vi "Тест_буфера_дублирвание_строк.vi"() -> ()   [LabVIEW 2013]
panel:
  out "Исходное сообщение":dbl[](array[numeric])
  in  "Кол-во копий":i32=5
  out "Подготовленный к отправке мажоритарный код":dbl[][](array[numeric])
  out "2-х массив на выходе 3":dbl[][](array[numeric])
  in  "Размер окна":i32=4
  out "Последовательность в массиве":dbl[](array[numeric])
  in  "Кол-во элементов":i32=16
  out "Array":dbl[][](array[numeric])
  in  "Размер окна буффера":i32
  out "Количество бит":i32
  in  "Количество бит":i32=8
  out "Биты на выходе":dbl[](array[numeric])
  # "3"
  # "15"
  # "7"
  # "3"
  # "7"
  # "15"
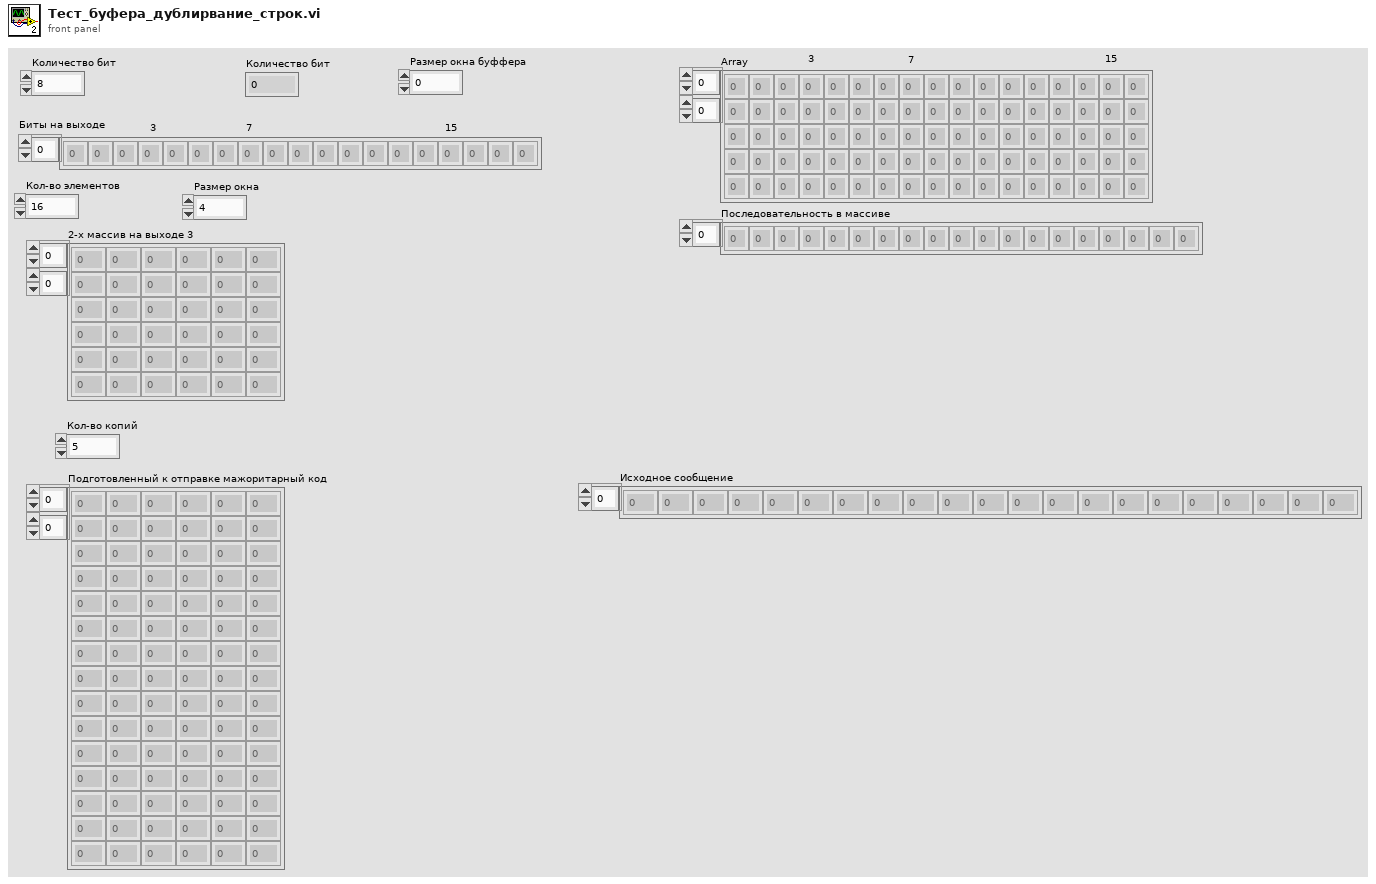
[diagram p1: front panel]
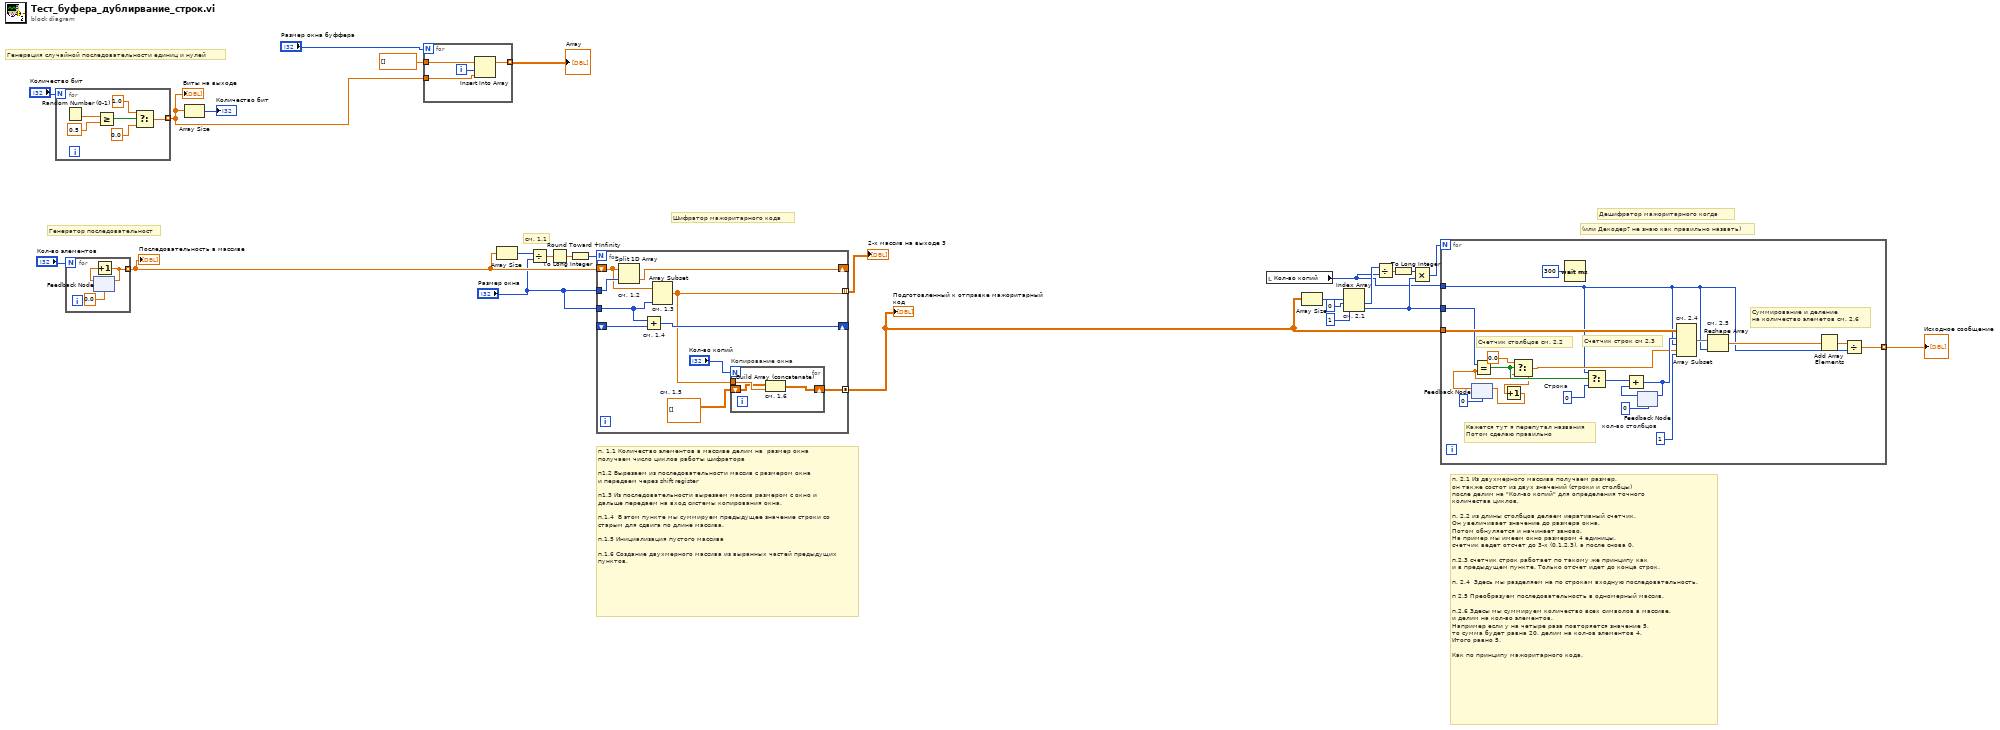
[diagram p0: block diagram]
diagram:
  # "п. 2.1 Из двухмерного массива получаем размер.\nон также состот из двух значений (строки и столбцы) \nпосле делим на \"Кол-во копий\" для определения точного\nколичества циклов.\n\nп. 2.2 из длины столбцов делаем иеративный счетчик. \nОн увеличивает значение до размера окна.\nПотом обнуляется и начинает заново.\nНа пример мы имеем окно размером 4 единицы.\nсчетчик ведет отсчет до 3-х (0,1,2,3), а после снова 0.\n\nп.2.3 счетчик строк работает по такому же принципу как \nи в предыдущем пункте. Только отсчет идет до конца строк.\n\nп. 2.4  Здесь мы разделяем на по строкам входную последовательность.\n\nп 2.5 Преобразуем последовательность в одномерный массив.\n\nп.2.6 Здесы мы суммируем количество всех символов в массиве.\nи делим на кол-во элементов.\nНапример если у на четыре раза повторяется значение 5, \nто сумма будет равна 20, делим на кол-ов элементов 4. \nИтого равно 5. \n\nКак по принципу мажоритарного кода."
  # "п. 1.1 Количество элементов в массиве делим на  размер окна\nполучаем число циклов работы шифратора\n\nп1.2 Вырезаем из последовательности массив с размером окна \nи передаем через shift register\n\nп1.3 Из последовательности вырезаем массив размером с окно и \nдальше передаем на вход системы копирования окна.\n \nп.1.4  В этом пункте мы суммируем предыдущее значение строки со\nстарым для сдвига по длине массива.\n\nп.1.5 Инициализация пустого массива\n\nп.1.6 Создание двухмерного массива из выранных частей предыдущих\nпунктов."
  # "см. 1.1"
  # "(или Декодер? не знаю как правильно назвать)"
  # "Дешифратор мажоритарного когда"
  # "Шифратор мажоритарного кода"
  # "Генератор последовательност"
  # "Генерация случайной последовательности единиц и нулей"
  n1 = for {
    N: "Количество бит" -> [_]
    tunnel: [w26] -> w20 mode=indexing
    n2 = Random Number (0-1)() -> (number: 0 to 1=w31:dbl)
    n3 = Greater Or Equal?(x=w31, y=0.5) -> (x >= y?=w29:bool)
    n4 = Select(t=1.0, s=w29, f=0.0) -> (s? t:f=w26:dbl)
  }
  "Биты на выходе" <- w20
  n5 = for {
    N: "Кол-во элементов" -> [_]
    tunnel: [w32] -> w17 mode=indexing
    n6 = feedback #1(0.0) -> (w34:dbl)
    n7 = Increment(x=w34) -> (x+1=w32:dbl)
    n8 = feedback-in #1(w32) -> ()
  }
  "Последовательность в массиве" <- w17
  n9 = Array Size(array=w20) -> (size(s)=→"Количество бит":i32)
  n10 = for {
    N: "Размер окна буффера" -> [_]
    tunnel: w20 -> [w36]
    tunnel: dbl[] [] -> [w37]
    tunnel: [w38] -> w23 mode=indexing
    i -> [w35]
    n11 = Insert Into Array(array=w37, index=w35, new element=w36) -> (w38:dbl[])
  }
  "Array" <- w23
  n12 = Array Size(array=w17) -> (size(s)=w18:i32)
  n13 = Divide(x=w18, y="Размер окна") -> (x/y=w16:dbl)
  n14 = Round Toward +Infinity(x=w16) -> (ceil(x): smallest int >= x=w15:dbl)
  n15 = To Long Integer(number=w15) -> (32bit integer=w12:i32)
  n16 = for {
    N: w12 -> [_]
    shift-right: [w48] -> _
    shift-left: w17 -> [w46]
    tunnel: "Размер окна" -> [w47]
    shift-right: [w44] -> _
    shift-left: _ -> [w43]
    tunnel: "Размер окна" -> [w45]
    tunnel: [w41] -> w13 mode=indexing
    tunnel: [w40] -> w8 mode=concatenating
    w39 = dbl[][] []  # см. 1.5
    n17 = Split 1D Array "см. 1.2"(array=w46, index=w47) -> (second subarray=w48:dbl[])  [unwired: 1 out]
    n18 = Add "см. 1.4"(x=w45, y=w43) -> (x+y=w44:i32)
    n19 = Array Subset "см. 1.3"(array=w46, length=w45) -> (w41:dbl[])  [unwired: 1 in]
    n20 = for "Копирование окна" {
      N: "Кол-во копий" -> [_]
      tunnel: w41 -> [w50]
      shift-right: [w51] -> w40
      shift-left: w39 -> [w49]
      n21 = Build Array (concatenate) "см. 1.6"(w49, w50) -> (w51:dbl[][])
    }
  }
  "2-х массив на выходе 3" <- w13
  "Подготовленный к отправке мажоритарный код" <- w8
  n22 = local read "Кол-во копий"() -> (w2:i32)
  n23 = Array Size(array=w8) -> (size(s)=w11:i32[])
  n24 = Index Array "см. 2.1"(array=w11, index #1=0 ("index"), index #2=1 ("index")) -> (element #1=w7:i32, element #2=w6:i32)
  n25 = Divide(x=w7, y=w2) -> (x/y=w5:dbl)
  n26 = To Long Integer(number=w5) -> (32bit integer=w4:i32)
  n27 = Multiply(x=w4, y=w6) -> (x*y=w3:i32)
  n28 = for {
    N: w3 -> [_]
    tunnel: w8 -> [w70]
    tunnel: w6 -> [w62]
    tunnel: w2 -> [w53]
    tunnel: [w52] -> w1 mode=indexing
    w69 = 1  # кол-во столбцов
    w60 = 0  # Строка
    # "Суммирование и деление \nна количество элеметов см. 2.6"
    # "Кажется тут я перепутал названия  \nПотом сделаю правильно"
    # "Счетчик строк см 2.3"
    # "Счетчик столбцов см. 2.2"
    n29 = feedback #2(0) -> (w58:dbl)
    n30 = Equal?(x=w62, y=w58) -> (x = y?=w64:bool)
    n31 = Select(t=0.0, s=w64, f=w58) -> (s? t:f=w57:dbl)
    n32 = Increment(x=w57) -> (x+1=w56:dbl)
    n33 = feedback-in #2(w56) -> ()
    n34 = Wait (ms)(milliseconds to wait=u32 300) -> ()  [unwired: 1 out]
    n35 = Select(t=w53, s=w64, f=w60) -> (s? t:f=w61:i32)
    n36 = feedback #3(0) -> (w63:i32)
    n37 = Add(x=w61, y=w63) -> (x+y=w59:i32)
    n38 = feedback-in #3(w59) -> ()
    n39 = Array Subset "см. 2.4"(array=w70, index (row)=w59, length (row)=w53, index (col)=w57, length (col)=w69) -> (w71:dbl[][])
    n40 = Reshape Array "см. 2.5"(w71, w53) -> (w55:dbl[])
    n41 = Add Array Elements(numeric array=w55) -> (sum=w54:dbl)
    n42 = Divide(x=w54, y=w53) -> (x/y=w52:dbl)
  }
  "Исходное сообщение" <- w1
